vi "Process Filled Buffer.vi"(8 "error in (no error)":errorcluster, 10 "Filled Buffers":T1, 11 "DAQ Interface in":refnum<class "DAQ Interface.lvclass">) -> (0 "error out":errorcluster, 3 "DAQ Interface out":refnum<class "DAQ Interface.lvclass">)   [LabVIEW 2025, in "DAQ Interface.lvlib" / "DAQ Interface.lvclass"]
uses:
  DAQ Interface.lvclass
  TDMS DAQ/TDMS DAQ/Filled Buffers.ctl
  <vilib>/Natan Biesmans/G2CPU GPU and CPU HPC Toolkit/G2CPU Libraries/Async IO/DMA Manager/DMA Manager.lvclass
  Signal Analysis/Signal Analysis/Process Data.ctl
  <vilib>/Natan Biesmans/G2CPU GPU and CPU HPC Toolkit/G2CPU Libraries/Arrays/1DArray/s16/1D Array s16.lvclass
  <vilib>/ActorFramework/Actor/Actor.lvclass/Actor.ctl
  <vilib>/ActorFramework/Message Enqueuer/Message Enqueuer.lvclass/Message Enqueuer.ctl
  DAQ Interface Messages/Return Available Buffer Msg/Return Available Buffer Msg.lvclass/Return Available Buffer Msg.ctl
  43816b8e-f5f8-4060-a8c5-425bb0051513.vi
  <vilib>/ActorFramework/Message Enqueuer/Init from Existing Queue.vi
  43816b8e-f5f8-4060-a8c5-425bb0051513.vi/67bb9abe-6be7-467c-be3d-dc59a1f5a88b.vi
  43816b8e-f5f8-4060-a8c5-425bb0051513.vi/bc198a8f-250c-4fb0-95cf-f9e16e559b40.vi
  43816b8e-f5f8-4060-a8c5-425bb0051513.vi/206e65cf-1cd8-4fd2-b98d-94b74801007d.vi
  <vilib>/ActorFramework/Message Enqueuer/Enqueue.vi
  DAQ Interface Messages/Return Available Buffer Msg/Return Available Buffer Msg.lvclass
  <vilib>/Natan Biesmans/G2CPU GPU and CPU HPC Toolkit/G2CPU Libraries/Manage Environment/G2CPU Get Backend.vi
  <vilib>/Utility/error.llb/Error Cluster From Error Code.vi
  <vilib>/Natan Biesmans/G2CPU GPU and CPU HPC Toolkit/ArrayFire Driver/VIs/Run as Multi Device.vi
  <vilib>/Natan Biesmans/G2CPU GPU and CPU HPC Toolkit/G2CPU Libraries/Async IO/CUDA Context FGV.vi
  <vilib>/Natan Biesmans/G2CPU GPU and CPU HPC Toolkit/G2CPU Libraries/Manage Environment/Find AF DLL.vi
  <vilib>/Natan Biesmans/G2CPU GPU and CPU HPC Toolkit/G2CPU Libraries/Arrays/Array/G2CPU Get Array Pointer.vi
  <vilib>/Natan Biesmans/G2CPU GPU and CPU HPC Toolkit/G2CPU Libraries/Arrays/Array/G2CPU Set Array Pointer.vi
  <vilib>/Natan Biesmans/G2CPU GPU and CPU HPC Toolkit/ArrayFire Driver/VIs/copy array.vi
  <vilib>/ActorFramework/Message Priority Queue/Priority Enqueue.vi
  <vilib>/ActorFramework/Message Enqueuer/Message Enqueuer.lvclass
  <vilib>/Natan Biesmans/G2CPU GPU and CPU HPC Toolkit/G2CPU Libraries/Arrays/Array/Array Prototype.lvclass
  DAQ Interface.lvclass/DAQ Interface.ctl
  <vilib>/ActorFramework/Actor/Actor.lvclass
  Signal Analysis/Signal Analysis/Signal Analysis.lvclass
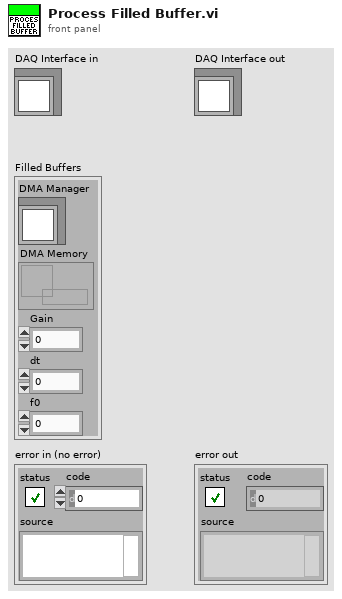
[diagram p1: front panel]
types:
  T1 = typedef "DAQ Interface.lvlib/DAQ Interface.lvclass/Filled Buffers.ctl" = cluster{"DMA Manager":refnum<class "DMA Manager.lvclass">, "DMA Memory":refnum<data-value>, "Gain":dbl, "dt":dbl, "f0":dbl}
  T2 = typedef "Signal Analysis.lvlib/Signal Analysis.lvclass/Process Data.ctl" = cluster{"Gain":dbl, "dt":dbl, "Serial IQ Data":refnum<class "1D Array s16.lvclass">, "f0":dbl}
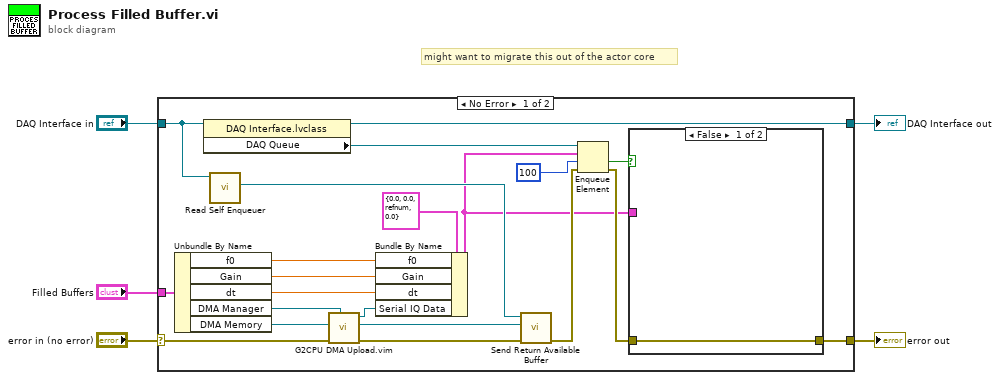
[diagram p0: block diagram]
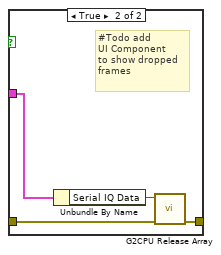
[diagram p2: hidden frame]
diagram:
  # "might want to migrate this out of the actor core"
  n1 = case shown="No Error" "error in (no error)" {
    selector: "error in (no error)" -> [w24 w33]
    tunnel: [w10 w33] -> w4
    tunnel: [w7 w32] -> w2
    tunnel: "DAQ Interface in" -> [w19 w32]
    tunnel: "Filled Buffers" -> [w26 _]
    frame No Error {
      n2 = Unbundle By Name(w26) -> ("f0"=w6:dbl, "Gain"=w13:dbl, "dt"=w12:dbl, "DMA Manager"=w25:refnum<class "DMA Manager.lvclass">, "DMA Memory"=w23:refnum<data-value>)
      n3 = property class="DAQ Interface.lvclass"(reference=w19) -> (reference out=w7:refnum<class "DAQ Interface.lvclass">, "DAQ Queue"=w18:refnum<queue>)  [unwired: 1 in, 1 out]
      n4 = call <vilib>:"Read Self Enqueuer.vi"("Actor"=w19) -> ("Self Enqueuer"=w20:refnum<class "Message Enqueuer.lvclass">)  [unwired: 10 in]
      n5 = call "G2CPU DMA Upload.vim"("DMA Manager"=w25, "error in (no error)"=w24, "Data In"=w23) -> ("error out"=w21:errorcluster, "Data Out"=w22:refnum<data-value>, "Array out"=w14:refnum<class "1D Array s16.lvclass">)  [unwired: 6 in]
      n6 = Bundle By Name(cluster=T2 {"Gain"=0.0, "dt"=0.0, "Serial IQ Data"=refnum, "f0"=0.0} ("element"), "f0"=w6, "Gain"=w13, "dt"=w12, "Serial IQ Data"=w14) -> (w8:T2)
      n7 = call "Send Return Available Buffer.vi"("error in (no error)"=w21, "DMA Memory"=w22, "Message Enqueuer"=w20) -> ("error out"=w17:errorcluster)  [unwired: 7 in, 1 out]
      n8 = Enqueue Element(queue=w18, element=w8, timeout in ms (-1)=100, error in (no error)=w17) -> (timed out?=w11:bool, error out=w9:errorcluster)  [unwired: 1 out]
      n9 = case shown="False" w11 {
        tunnel: [w27 w30] -> w10
        tunnel: w9 -> [w27 w31]
        tunnel: w8 -> [_ w29]
        frame False {
        }
        frame True {
          # "#Todo add \nUI Component\nto show dropped\nframes"
          n10 = Unbundle By Name(w29) -> ("Serial IQ Data"=w28:refnum<class "1D Array s16.lvclass">)
          n11 = call <vilib>:"G2CPU Release Array.vi"("error in (no error)"=w31, "Array in"=w28) -> ("error out"=w30:errorcluster)  [unwired: 9 in]
        }
      }
    }
    frame Error {
    }
  }
  "error out" <- w4
  "DAQ Interface out" <- w2
